vi "Breakdown manage1.vi"(8 "error in (no error)":errorcluster) -> ()   [LabVIEW 2017]
uses:
  <vilib>/Utility/miscctls.llb/LVRowAndColumnTypeDef.ctl
  <vilib>/addons/database/Connection.llb/DB Tools Open Connec (Path).vi
  <vilib>/Utility/file.llb/Write Delimited Spreadsheet (string).vi
  <vilib>/addons/database/NI_Database_API.lvlib
panel:
  in  "Back 2":bool
  in  "Download 2":bool
  in  "Get Rport":bool
  in  "Manage":bool
  out "Table":string[][](table)
  out "Run-Time Status":cluster{"Array 2":timestamp[], dbl[]}(graph)
  out "subarray":string[](array[string])
  in  "Export to Excel":bool
  in  "Shift":string(combo)
  out "error out":errorcluster
  in  "Select Line":string(combo)
  in  "To Date":timestamp format="%<%Y-%m-%d>T"
  in  "Form Date":timestamp format="%<%Y-%m-%d>T"
  in  "Delete":bool
  in  "Edit":bool
  in  "Select Stakeholder":string(combo)
  in  "Get Report":bool
  # "Breakdown Manage"
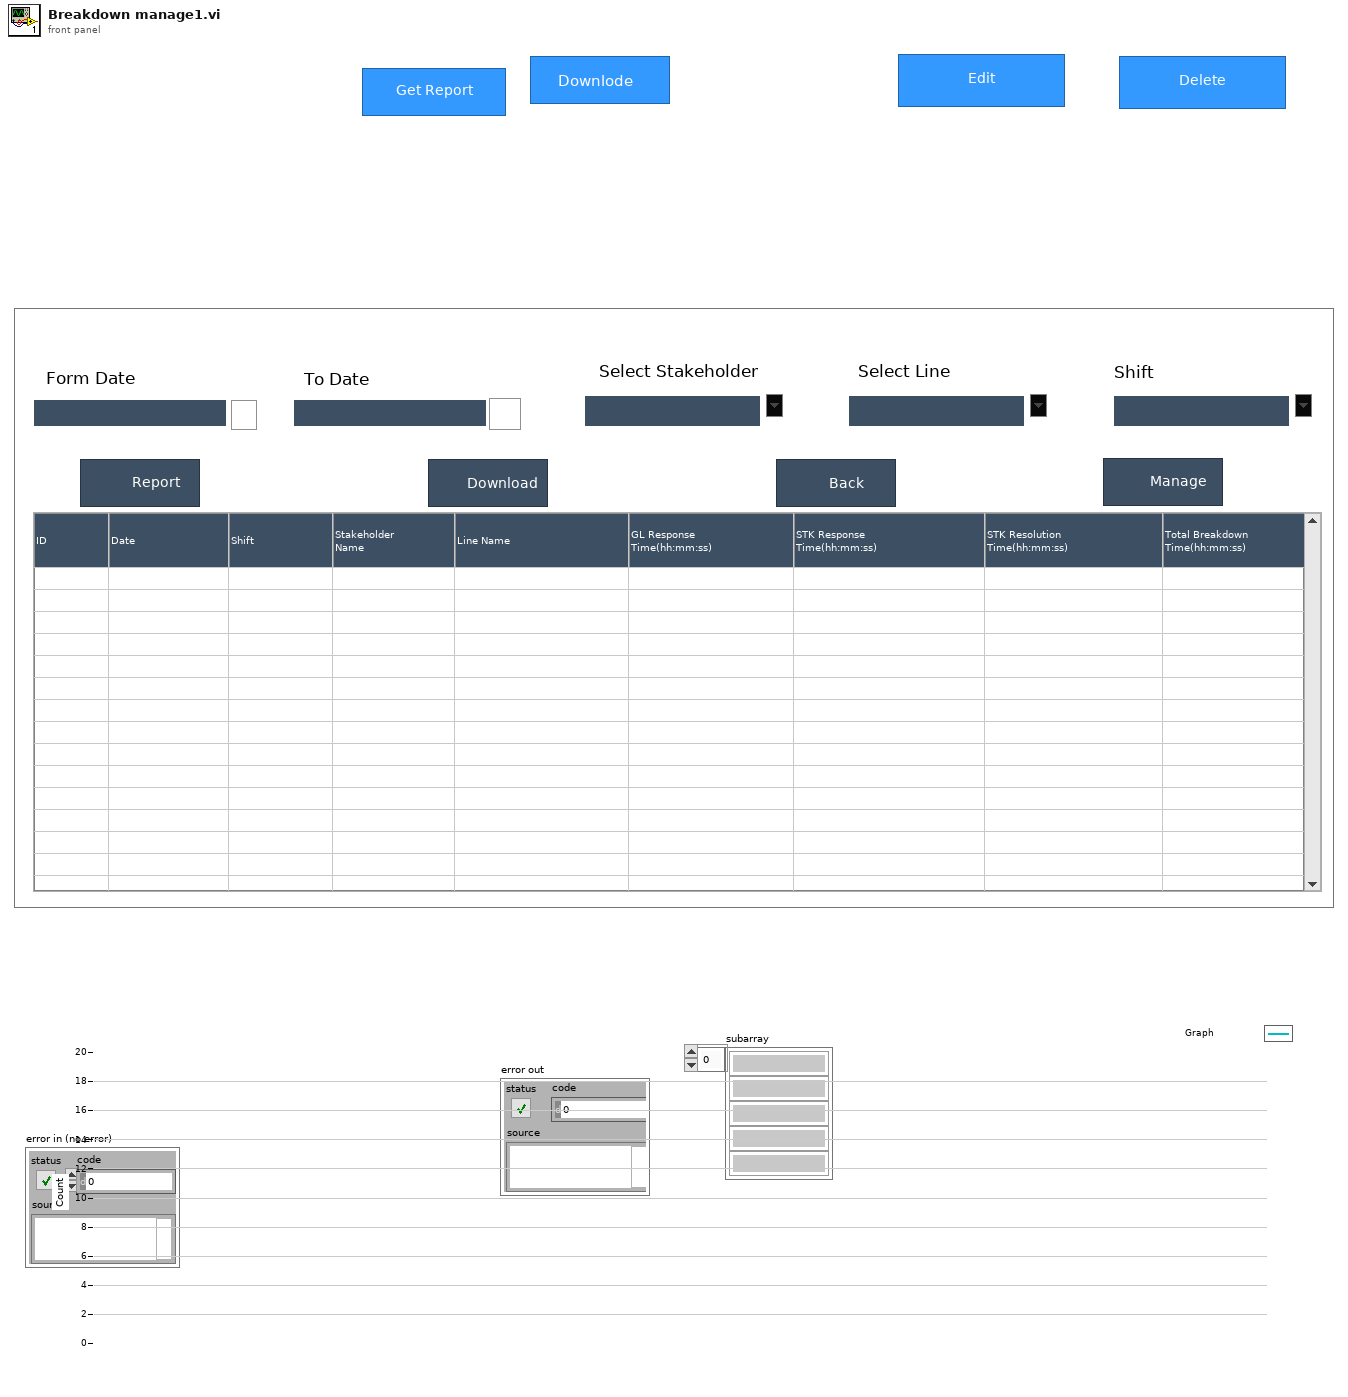
[diagram p1: front panel]
types:
  T1 = typedef "LVRowAndColumnTypeDef.ctl" = cluster{"Row":i32, "Column":i32}
  T2 = typedef "NI_Database_API.lvlib/Conn ObjectReference.ctl" = refnum<k1>
  T3 = enum32{"invalid app kind", "Development System", "Run Time System", "Student Edition", "Embedded LabVIEW", "Evaluation", "Custom"}
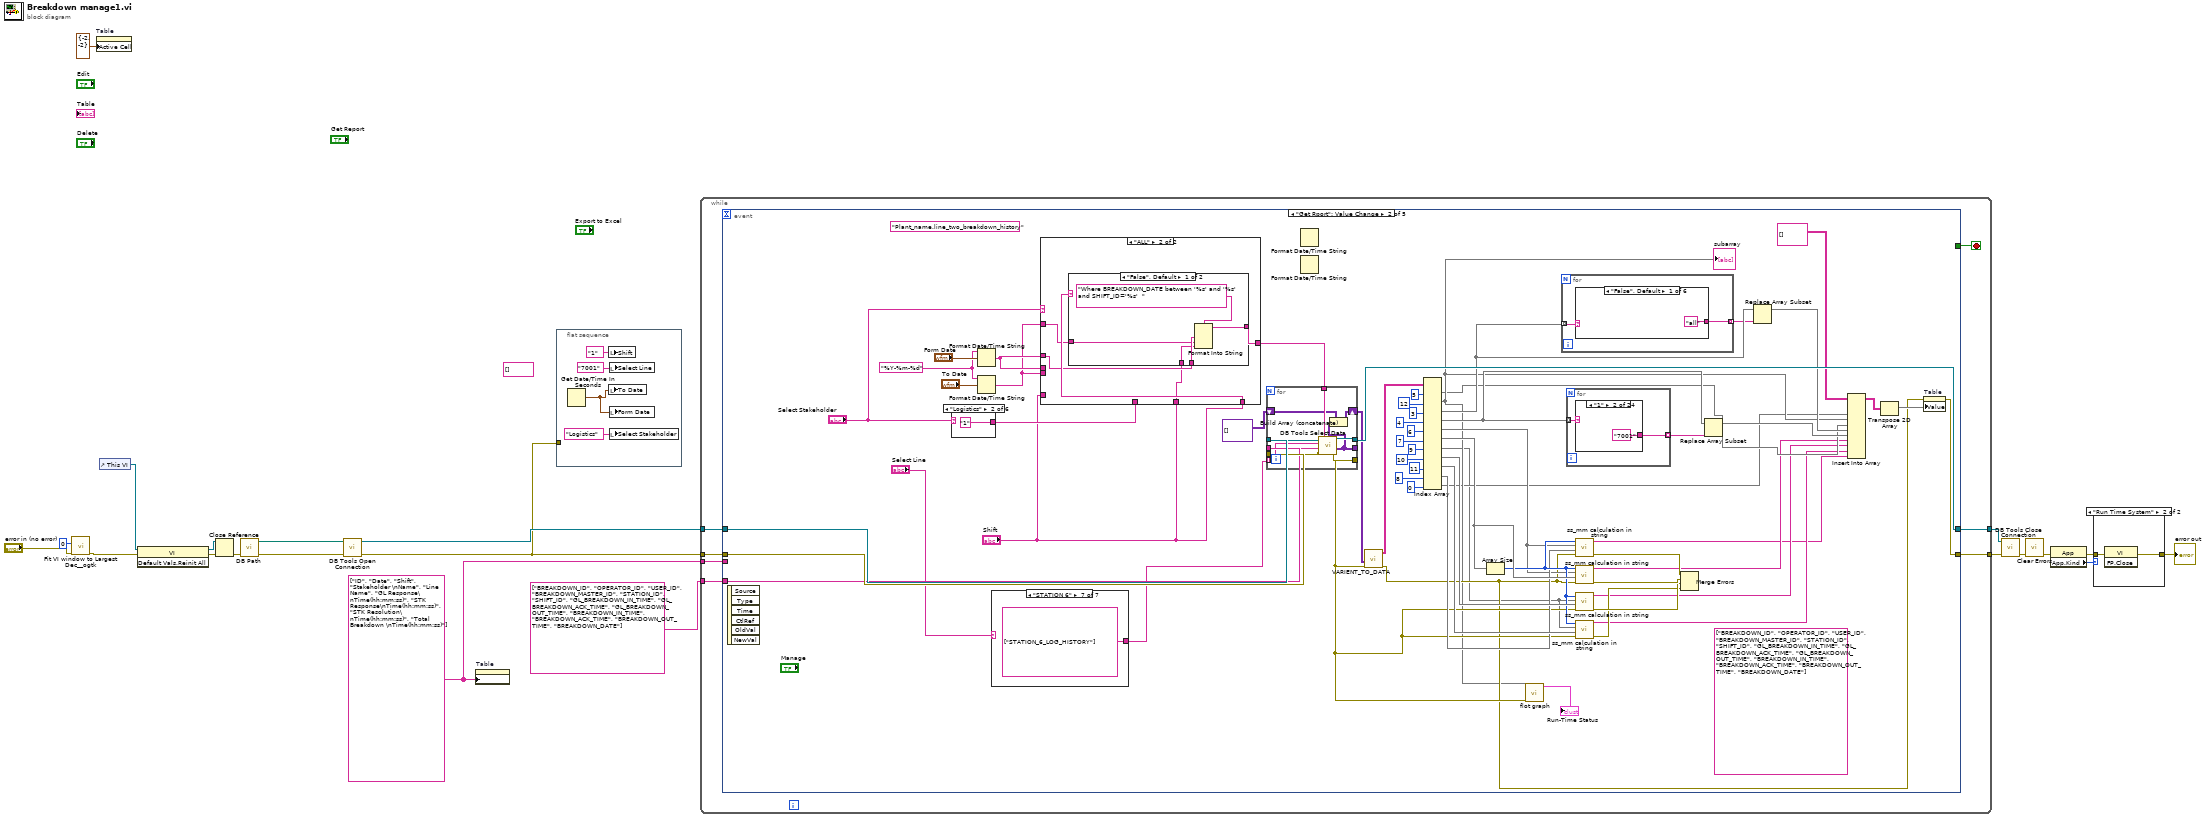
[diagram p0: block diagram]
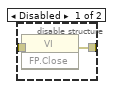
[diagram p3: hidden frame]
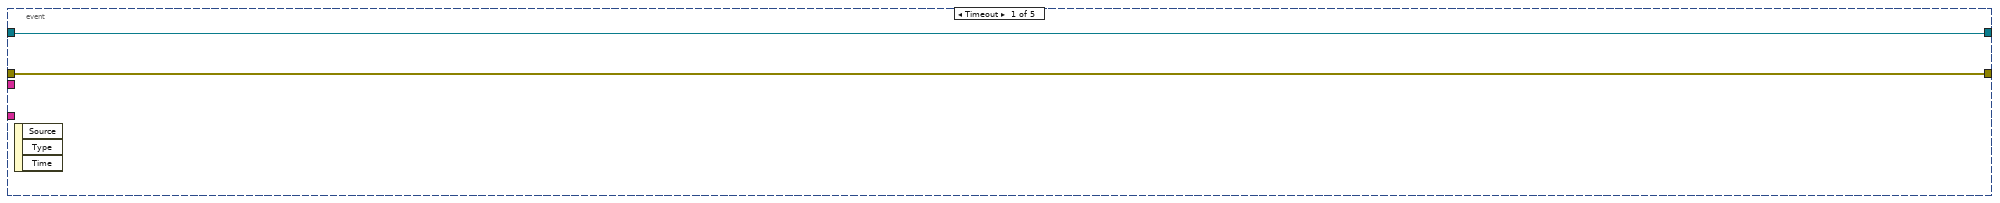
[diagram p4: hidden frame]
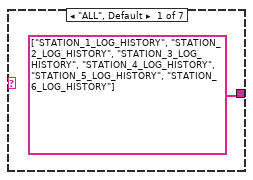
[diagram p5: hidden frame]
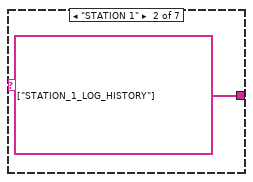
[diagram p6: hidden frame]
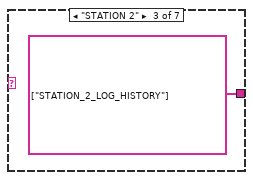
[diagram p7: hidden frame]
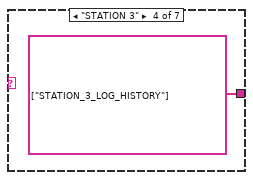
[diagram p8: hidden frame]
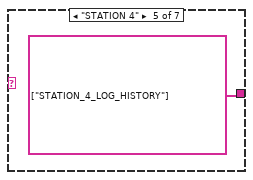
[diagram p9: hidden frame]
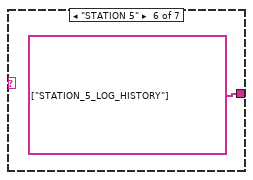
[diagram p10: hidden frame]
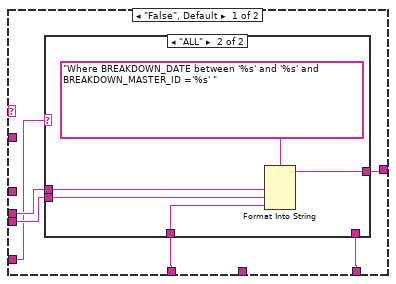
[diagram p11: hidden frame]
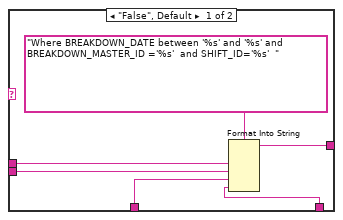
[diagram p12: hidden frame]
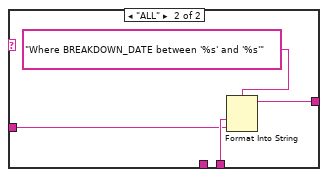
[diagram p13: hidden frame]
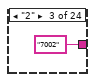
[diagram p15: hidden frame]
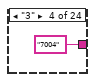
[diagram p16: hidden frame]
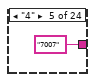
[diagram p17: hidden frame]
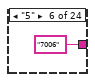
[diagram p18: hidden frame]
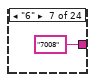
[diagram p19: hidden frame]
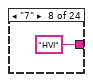
[diagram p20: hidden frame]
diagram:
  (unwired) string[] []
  w5 = string[] ["ID", "Date", "Shift", "Stakeholder \nName", "Line Name", "GL Response\nTime(hh:mm:ss)", "STK Response\nTime(hh:mm:ss)", "STK Resolution\nTime(hh:mm:ss)", "Total Breakdown \nTime(hh:mm:ss)"] ("Column Header Strings[]")
  n1 = call <userlib>:"Fit VI window to Largest Dec__ogtk.vi"("error in (no error)"="error in (no error)", "border spacing (2 px)"=0) -> ("error out"=w3:errorcluster)  [unwired: 4 in, 1 out]
  n2 = property on="Table" class="Tbl (strict)"("Active Cell"=T1 {"Row"=-2, "Column"=-2} ("Active Cell:Active Cell")) -> ()  [unwired: 2 in, 2 out]
  n3 = control-ref of="This VI"() -> (w20:refnum<vi>)
  n4 = invoke class="VI" method="Default Vals.Reinit All"(reference=w20, error in=w3) -> (reference out=w18:refnum<vi>, error out=w19:errorcluster)  [unwired: 1 in, 1 out]
  n5 = Close Reference(reference=w18, error in (no error)=w19) -> (error out=w11:errorcluster)
  n6 = call "DB Path.vi"("error in"=w11) -> ("error out"=w10:errorcluster, "DB Path"=w9:path)  [unwired: 9 in]
  n7 = call-poly <vilib>:"DB Tools Open Connection.vi"("error in (no error)"=w10, "connection information"=w9) -> ("error out"=w1:errorcluster, "connection reference"=w8:T2)  [unwired: 6 in]
  n8 = property on="Table" class="Tbl (strict)"("Column Headers[]"=w5) -> ()  [unwired: 2 in, 2 out]
  n9 = flat-sequence {
    tunnel: w1 -> [_]
    frame #0 {
      n10 = Get Date/Time In Seconds() -> (seconds since 1Jan1904=w25:timestamp)
      n11 = local write "Shift"("1" ("Shift")) -> ()
      n12 = local write "To Date"(w25) -> ()
      n13 = local write "Select Line"("7001" ("Select Line")) -> ()
      n14 = local write "Form Date"(w25) -> ()
      n15 = local write "Select Stakeholder"("Logistics" ("Select Stakeholder")) -> ()
    }
  }
  n16 = while {
    tunnel: w1 -> [w32]
    tunnel: [w31] -> w14
    tunnel: [w29] -> w12
    tunnel: w8 -> [w28]
    tunnel: string[] ["BREAKDOWN_ID", "OPERATOR_ID", "USER_ID", "BREAKDOWN_MASTER_ID", "STATION_ID", "SHIFT_ID", "GL_BREAKDOWN_IN_TIME", "GL_BREAKDOWN_ACK_TIME", "GL_BREAKDOWN_OUT_TIME", "BREAKDOWN_IN_TIME", "BREAKDOWN_ACK_TIME", "BREAKDOWN_OUT_TIME", "BREAKDOWN_DATE"] ("columns") -> [w27]
    tunnel: w5 -> [w26]
    stop <- w30 stop-if-true
    n17 = event shown="[1] \"Get Rport\": Value Change" {
      selector: _ -> [_ _ _ _ _]
      dyn-events: _ -> [_ _ _ _ _]
      timeout: _ -> [_ _ _ _ _]
      tunnel: w32 -> [w34 w92 w182 w187 _]
      tunnel: [w34 w61 w181 w186 _] -> w31
      tunnel: [_ _ _ _ TRUE] -> w30
      tunnel: [w33 w93 _ _ _] -> w29
      tunnel: w28 -> [w33 w94 _ _ _]
      tunnel: w27 -> [_ w89 _ _ _]
      tunnel: w26 -> [_ _ _ _ _]
      event Timeout {
        n18 = event-data() -> ()  [unwired: 1 in, 3 out]
      }
      event "Get Rport": Value Change {
        (unwired) string[] ["BREAKDOWN_ID", "OPERATOR_ID", "USER_ID", "BREAKDOWN_MASTER_ID", "STATION_ID", "SHIFT_ID", "GL_BREAKDOWN_IN_TIME", "GL_BREAKDOWN_ACK_TIME", "GL_BREAKDOWN_OUT_TIME", "BREAKDOWN_IN_TIME", "BREAKDOWN_ACK_TIME", "BREAKDOWN_OUT_TIME", "BREAKDOWN_DATE"] ("columns")
        (unwired) "Plant_name.line_two_breakdown_history" ("table")
        w87 = "%Y-%m-%d" ("time format string (%c)")
        n19 = event-data() -> ()  [unwired: 1 in, 6 out]
        n20 = case shown="\"Logistics\"" "Select Stakeholder" {
          tunnel: [_ "1" "2" "3" "4" "5"] -> w88
          frame "False", Default {
          }
          frame "Logistics" {
          }
          frame "Maintenance" {
          }
          frame "Quality" {
          }
          frame "Production" {
          }
          frame "Gap Leader" {
          }
        }
        n21 = Format Date/Time String(time format string (%c)=w87, seconds (now)="Form Date") -> (date/time string=w57:string)  [unwired: 1 in]
        n22 = Format Date/Time String(time format string (%c)=w87, seconds (now)="To Date") -> (date/time string=w56:string)  [unwired: 1 in]
        n23 = case shown="\"STATION 6\"" "Select Line" {
          tunnel: [string[] ["STATION_1_LOG_HISTORY", "STATION_2_LOG_HISTORY", "STATION_3_LOG_HISTORY", "STATION_4_LOG_HISTORY", "STATION_5_LOG_HISTORY", "STATION_6_LOG_HISTORY"] string[] ["STATION_1_LOG_HISTORY"] string[] ["STATION_2_LOG_HISTORY"] string[] ["STATION_3_LOG_HISTORY"] string[] ["STATION_4_LOG_HISTORY"] string[] ["STATION_5_LOG_HISTORY"] string[] ["STATION_6_LOG_HISTORY"]] -> w36
          frame "ALL", Default {
          }
          frame "STATION 1" {
          }
          frame "STATION 2" {
          }
          frame "STATION 3" {
          }
          frame "STATION 4" {
          }
          frame "STATION 5" {
          }
          frame "STATION 6" {
          }
        }
        n24 = case shown="\"ALL\"" "Select Stakeholder" {
          tunnel: [w112 w129] -> w54
          tunnel: w57 -> [w117 _]
          tunnel: w56 -> [w116 _]
          tunnel: w88 -> [w115 _]
          tunnel: "Shift" -> [w114 w133]
          tunnel: "Shift" -> [w113 _]
          tunnel: w57 -> [_ w132]
          tunnel: w56 -> [_ w131]
          tunnel: "Shift" -> [_ w130]
          frame "False", Default {
            n25 = case shown="\"ALL\"" w113 {
              tunnel: [w122 w127] -> w112
              tunnel: w117 -> [w121 w126]
              tunnel: w116 -> [w120 w125]
              tunnel: w115 -> [w119 w124]
              tunnel: w114 -> [w118 _]
              frame "False", Default {
                n26 = Format Into String(format string="Where BREAKDOWN_DATE between '%s' and '%s' and BREAKDOWN_MASTER_ID ='%s'  and SHIFT_ID='%s'  " ("condition"), w121, w120, w119, w118) -> (resulting string=w122:string)  [unwired: 2 in, 1 out]
              }
              frame "ALL" {
                n27 = Format Into String(format string="Where BREAKDOWN_DATE between '%s' and '%s' and BREAKDOWN_MASTER_ID ='%s' " ("condition"), w126, w125, w124) -> (resulting string=w127:string)  [unwired: 2 in, 1 out]
              }
            }
          }
          frame "ALL" {
            n28 = case shown="\"False\", Default" w133 {
              tunnel: w132 -> [w137 w141]
              tunnel: w131 -> [w136 w140]
              tunnel: w130 -> [w135 _]
              tunnel: [w134 w139] -> w129
              frame "False", Default {
                n29 = Format Into String(format string="Where BREAKDOWN_DATE between '%s' and '%s' and SHIFT_ID='%s'  " ("condition"), w137, w136, w135) -> (resulting string=w134:string)  [unwired: 2 in, 1 out]
              }
              frame "ALL" {
                n30 = Format Into String(format string="Where BREAKDOWN_DATE between '%s' and '%s'" ("condition"), w141, w140) -> (resulting string=w139:string)  [unwired: 2 in, 1 out]
              }
            }
          }
        }
        n31 = for {
          tunnel: w36 -> [w109] mode=indexing
          tunnel: [w103] -> _
          tunnel: w89 -> [w105]
          tunnel: w54 -> [w106]
          tunnel: w92 -> [w108]
          tunnel: [w107] -> w60
          tunnel: w94 -> [w111]
          tunnel: [w110] -> w93
          shift-right: [w102] -> w52
          shift-left: variant[][] [] ("data") -> [w104]
          n32 = call <vilib>:"DB Tools Select Data.vi"("condition"=w106, "error in (no error)"=w108, "columns"=w105, "table"=w109, "connection reference"=w111) -> ("error out"=w107:errorcluster, "data"=w103:variant[][], "connection reference out"=w110:T2)  [unwired: 1 in]
          n33 = Build Array (concatenate)(w104, w103) -> (w102:variant[][])
        }
        n34 = Format Date/Time String() -> ()  [unwired: 3 in, 1 out]
        n35 = Format Date/Time String() -> ()  [unwired: 3 in, 1 out]
        n36 = call "VARIENT_TO_DATA.vi"("data"=w52, "error in (no error)"=w60) -> ("Table"=w82:string[][], "error out"=w47:errorcluster)  [unwired: 7 in]
        n37 = Index Array(array=w82, index (col) #1=5 ("disabled index (col)"), index (col) #2=12 ("disabled index (col)"), index (col) #3=3 ("index (col)"), index (col) #4=4 ("index (col)"), index (col) #5=6 ("index (col)"), index (col) #6=7 ("index (col)"), index (col) #7=9 ("index (col)"), index (col) #8=10 ("index (col)"), index (col) #9=11 ("index (col)"), index (col) #10=8 ("index (col)"), index (col) #11=0 ("index (col)")) -> (element #1=w44:string[], element #2=w45:string[], element #3=w84:string[], element #4=w70:string[], element #5=w62:string[], element #6=w67:string[], element #7=w35:string[], element #8=w66:string[], element #9=w65:string[], element #10=w63:string[], element #11=w38:string[])  [unwired: 11 in]
        "subarray" <- w45
        n38 = Array Size(array=w67) -> (size(s)=w64:i32)
        n39 = call "flot graph.vi"("BD Date"=w45, "error in (no error)"=w60) -> ("Run-Time Status"=→"Run-Time Status":cluster{"Array 2":timestamp[], dbl[]})  [unwired: 9 in]
        n40 = for {
          tunnel: w84 -> [w169] mode=indexing
          tunnel: [w168] -> w83 mode=indexing
          n41 = case shown="\"False\", Default" w169 {
            tunnel: ["all" "Safety" "Logistics" "Maintenance" "Quality" "Production"] -> w168
            frame "False", Default {
            }
            frame "1" {
            }
            frame "2" {
            }
            frame "3" {
            }
            frame "4" {
            }
            frame "5" {
            }
          }
        }
        n42 = for {
          tunnel: w70 -> [w144] mode=indexing
          tunnel: [w143] -> w69 mode=indexing
          n43 = case shown="\"1\"" w144 {
            tunnel: [_ "7001" "7002" "7004" "7007" "7006" "7008" "HVI" "7009" "SA" "M&M" "TML" "5001" "1001" "4003" "1002" "4004" "1004" "2001" "3001" "2004" "3002" "3003" "4001"] -> w143
            frame "0", Default {
            }
            frame "1" {
            }
            frame "2" {
            }
            frame "3" {
            }
            frame "4" {
            }
            frame "5" {
            }
            frame "6" {
            }
            frame "7" {
            }
            frame "8" {
            }
            frame "9" {
            }
            frame "10" {
            }
            frame "11" {
            }
            frame "12" {
            }
            frame "13" {
            }
            frame "14" {
            }
            frame "15" {
            }
            frame "16" {
            }
            frame "17" {
            }
            frame "18" {
            }
            frame "19" {
            }
            frame "20" {
            }
            frame "21" {
            }
            frame "22" {
            }
            frame "23" {
            }
          }
        }
        n44 = call "ss_mm calculation in string.vi"("error in (no error)"=w47, "Table 2"=w63, "Table"=w62, "Numeric"=w64) -> ("error out"=w51:errorcluster, "Array 2"=w40:string[])  [unwired: 6 in]
        n45 = call "ss_mm calculation in string.vi"("error in (no error)"=w47, "Table 2"=w67, "Table"=w62, "Numeric"=w64) -> ("error out"=w50:errorcluster, "Array 2"=w43:string[])  [unwired: 6 in]
        n46 = call "ss_mm calculation in string.vi"("error in (no error)"=w60, "Table 2"=w66, "Table"=w35, "Numeric"=w64) -> ("error out"=w49:errorcluster, "Array 2"=w42:string[])  [unwired: 6 in]
        n47 = call "ss_mm calculation in string.vi"("error in (no error)"=w60, "Table 2"=w65, "Table"=w35, "Numeric"=w64) -> ("error out"=w48:errorcluster, "Array 2"=w41:string[])  [unwired: 6 in]
        n48 = Merge Errors(w51, w50, w49, w48) -> ()  [unwired: 1 out]
        n49 = Replace Array Subset(array=w70, new element=w69) -> (w68:string[])  [unwired: 1 in]
        n50 = Replace Array Subset(array=w84, new element=w83) -> (w80:string[])  [unwired: 1 in]
        n51 = Insert Into Array(array=string[][] [], new element #1=w38, new element #2=w45, new element #3=w44, new element #4=w80, new element #5=w68, new element #6=w43, new element #7=w42, new element #8=w41, new element #9=w40) -> (w79:string[][])  [unwired: 2 in]
        n52 = Transpose 2D Array(2D array=w79) -> (transposed array=w78:string[][])
        n53 = property on="Table" class="Tbl (strict)"(error in=w47, "Value"=w78) -> (error out=w61:errorcluster)  [unwired: 1 in, 1 out]
      }
      event "Manage": Value Change {
        # "BREAKDOWN_STK_HOLD_ID"
        n54 = event-data() -> ()  [unwired: 1 in, 6 out]
        n55 = call "manage breakdown sub.vi"("error in (no error)"=w182) -> ("error out"=w181:errorcluster)  [unwired: 10 in]
      }
      event "Download 2": Value Change {
        n56 = event-data() -> ()  [unwired: 1 in, 6 out]
        n57 = call "File Dialog"() -> ("selected path"=w191:path, "error out"=w190:errorcluster)  [unwired: 12 in, 2 out]
        n58 = call <vilib>:"Clear Errors.vi"("error in (no error)"=w190) -> ()  [unwired: 5 in, 2 out]
        n59 = Path To String(path=w191) -> (string=w192:string)
        n60 = Concatenate Strings(w192, ".csv" ("string")) -> (w193:string)
        n61 = property on="Table" class="Tbl (strict)"() -> ("Value"=w188:string[][])  [unwired: 2 in, 2 out]
        n62 = String To Path(string=w193) -> (path=w194:path)
        n63 = Build Array (concatenate)(string[][] [["ID", "Date", "Shift", "Stakeholder Name", "Line Name", "GL Response Time", "STK Response Time(hh:mm:ss)", "STK Resolution Time(hh:mm:ss)", "Total Breakdown Time(hh:mm:ss)"]] ("Column Header Strings[]"), w188) -> (w183:string[][])
        n64 = call-poly <vilib>:"Write Delimited Spreadsheet.vi"("file path (dialog if empty)"=w194, "2D data"=w183, "error in (no error)"=w187, "delimiter (\\t)"="," ("delimiter (\\t)")) -> ("error out"=w186:errorcluster)  [unwired: 10 in, 1 out]
      }
      event "Back 2": Value Change {
        n65 = event-data() -> ()  [unwired: 1 in, 6 out]
      }
    }
  }
  n66 = call <vilib>:"DB Tools Close Connection.vi"("error in (no error)"=w14, "connection reference"=w12) -> ("error out"=w15:errorcluster)  [unwired: 5 in]
  n67 = call <vilib>:"Clear Errors.vi"("error in (no error)"=w15) -> ("error out"=w13:errorcluster)  [unwired: 5 in, 1 out]
  n68 = property class="App"(error in=w13) -> (error out=w16:errorcluster, "App.Kind"=w17:T3)  [unwired: 1 in, 1 out]
  n69 = case shown="\"Run Time System\"" w17 {
    tunnel: w16 -> [w197 w202]
    tunnel: [w196 w201] -> w6
    frame Default {
      n70 = disable-structure shown="Enabled" {
        disable-tunnel: w197 -> [w199 w200]
        disable-tunnel: [w198 w200] -> w196
        frame Disabled {
          n71 = invoke class="VI" method="FP.Close"(error in=w199) -> (error out=w198:errorcluster)  [unwired: 2 in, 2 out]
        }
        frame Enabled {
        }
      }
    }
    frame "Run Time System" {
      n72 = invoke class="VI" method="FP.Close"(error in=w202) -> (error out=w201:errorcluster)  [unwired: 2 in, 2 out]
    }
  }
  "error out" <- w6
